vi "HitrapGUI.constructor.vi"(0 "name":string, 2 "data in":string, 5 "error in (no error)":errorcluster) -> (14 "i ref out":refnum<vi>, 16 "data out":string, 19 "error out":errorcluster)   [LabVIEW 2014, in "HitrapGUI.lvlib"]
doc: "This is the constructor of a class.\n\nLicense Agreement for this software:\n\nCopyright (C)\nGesellschaft für Schwerionenforschung, GSI\nPlanckstr. 1\n64291 Darmstadt\nGermany\n\nContact: D.Beck@gsi.de \n\nThis program is free software; you can redistribute it and/or modify it under the terms of the \nGNU General Public License as published by the Free Software Foundation; either version 2 of \nthe license, or (at your option) any later version.\n\nThis program is distributed in the hope that it will be useful, but WITHOUT ANY WARRANTY; \nwithout even the implied warranty of MERCHANTABILITY or FITNESS FOR A PARTICULAR PURPOSE. See the GNU General License for more details (http://www.gnu.org).\n\nGesellschaft für Schwerionenforschung, GSI\nPlanckstr. 1, 64291 Darmstadt, Germany\nFor all questions and ideas contact: M.Richter@gsi.de, H.Brand@gsi.de or D.Beck@gsi.de.\nLast update: 16-JUN-2004"
uses:
  HitrapGUI.lvlib
  CS_Core/CSSystem/CoreLib/CoreLib.byte array 2 string.vi
  CS_Core/GUIs/GOGControllerGUI/GOGControllerGUI.lvlib
  CS_Core/CSSystem/CSSystemLib/CSSystemLib.lvlib
  CS_Core/BaseProcess/BaseProcess.lvlib
  CS_Core/CSSystem/CoreLib/CoreLib.lvlib
  CSlibraries-extern/DimLVEvent/LVDimInterface/LVDimInterface.lvlib
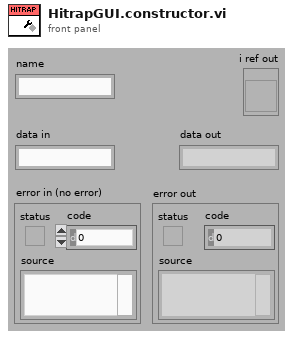
[diagram p1: front panel]
types:
  T1 = enum16{"SetAttribute", "GetAttribute", "CreateAttribute", "DestroyAttribute", "DestroyAllAtributes"}
  T2 = typedef "BaseProcess.lvlib/BaseProcess.i attribute.ctl" = cluster{"EventStatus":string, "EventError":i32, "PresetEvtWatchD":i32, "PresetPdcWatchD":i32, "EventTimeout":i32, "PeriodicInterval":i32, "Interface":string[], "Address":string[], "Special":string[], "PeriodicError":i32, "PeriodicStatus":string, "SuperProc":string, "Descriptors":T3[], "CaseRef":refnum<vi>, "PdcRef":refnum<vi>, "Thread Ref":refnum<vi>, "eventErrorID":i32, "eventStatusID":i32, "periodicErrorID":i32, "periodicStatusID":i32, "pdcCtrID":i32}
  T3 = typedef "BaseProcess.lvlib/BaseProcess.descriptor definition.ctl" = cluster{"selector":string, "descriptor":T4}
  T4 = typedef "BaseProcess.lvlib/BaseProcess.descriptor string definition.ctl" = string
  T5 = typedef "CoreDefs.call_type.ctl" = cluster{"Object":string, "Selector":string, "CallType":enum16{"simple", "synchronous", "asynchronous"}, "Async Object":string, "Async Selector":string, "Data Descriptor":T4, "Data":T6, "Error #":i32, "Expire":u32}
  T6 = typedef "CoreDefs.rawDataType.ctl" = i8[]
  T7 = typedef "HitrapGUI.lvlib/HitrapGUI.i attribute.ctl" = cluster{"SVs":refnum<k21>[], "DSCIntProc":string, "MotorActivityID":i32}
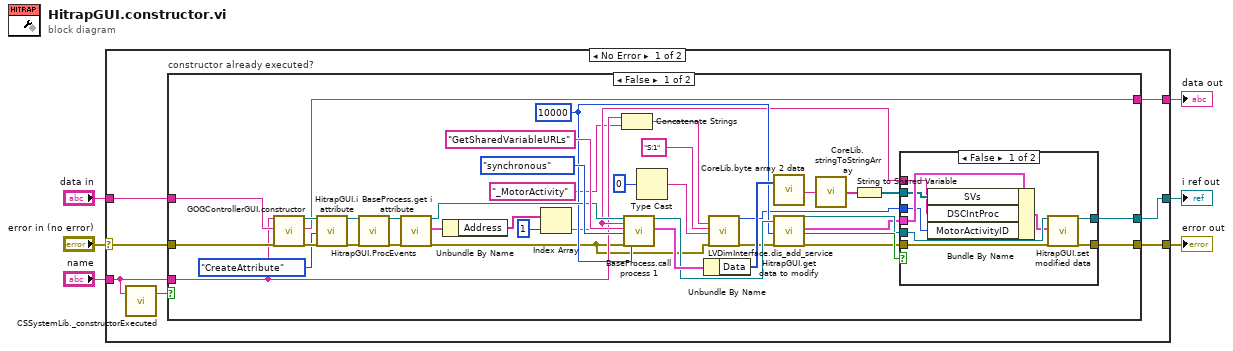
[diagram p0: block diagram]
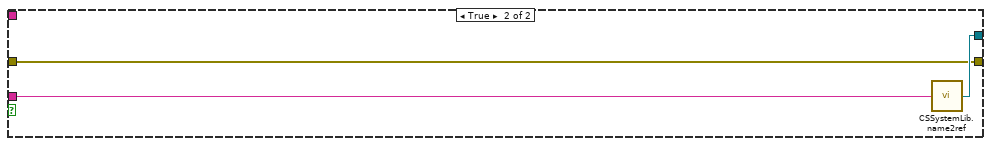
[diagram p3: hidden frame]
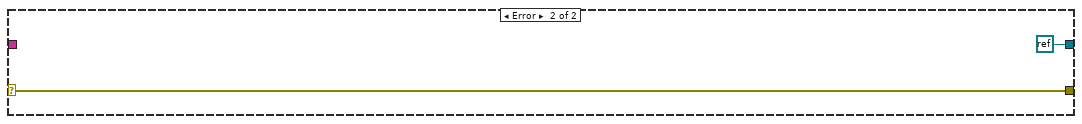
[diagram p4: hidden frame]
diagram:
  n1 = case shown="No Error" "error in (no error)" {
    selector: "error in (no error)" -> [w11 w67]
    tunnel: "name" -> [w10 _]
    tunnel: [w13 refnum<k0> refnum] -> w5
    tunnel: [w12 w67] -> w4
    tunnel: "data in" -> [w8 _]
    tunnel: [w7 _] -> w1
    frame No Error {
      n2 = call "CSSystemLib._constructorExecuted.vi"("name"=w10) -> ("constructor executed?"=w9:bool)  [unwired: 18 in]
      n3 = case "constructor already executed?" shown="False" w9 {
        tunnel: w10 -> [w19 w66]
        tunnel: [w29 w65] -> w13
        tunnel: [w27 w64] -> w12
        tunnel: w11 -> [w47 w64]
        tunnel: w8 -> [w46 _]
        tunnel: [w45 _] -> w7
        frame False {
          w32 = 10000 ("timeout (ms)")
          n4 = call "GOGControllerGUI.constructor.vi"("name"=w19, "data in"=w46, "error in (no error)"=w47) -> ("i ref out"=w52:refnum<vi>, "data out"=w45:string, "error out"=w51:errorcluster)  [unwired: 14 in]
          n5 = call "HitrapGUI.i attribute.vi"("VI Refnum"=w52, "Action"=T1."CreateAttribute", "error in (no error)"=w51) -> ("VI Refnum out"=w49:refnum<vi>, "error out"=w48:errorcluster)  [unwired: 14 in, 1 out]
          n6 = call "HitrapGUI.ProcEvents.vi"("i ref in"=w49, "error in (no error)"=w48) -> ("i ref out"=w34:refnum<vi>, "error out"=w35:errorcluster)  [unwired: 16 in]
          n7 = call "BaseProcess.get i attribute.vi"("i ref in"=w34, "error in (no error)"=w35) -> ("i ref out"=w36:refnum<vi>, "i attribute"=w44:T2, "error out"=w14:errorcluster)  [unwired: 15 in]
          n8 = Unbundle By Name(w44) -> ("Address"=w43:string[])
          n9 = Index Array(array=w43, index=1) -> (element=w23:string)
          n10 = Concatenate Strings(w19, "_MotorActivity" ("string")) -> (w20:string)
          n11 = call "BaseProcess.call process 1.vi"("i ref in"=w36, "Object"=w23, "Selector"="GetSharedVariableURLs", "CallType"=enum16{"simple", "synchronous", "asynchronous"}."synchronous", "error in (no error)"=w14, "timeout (ms)"=w32) -> ("i ref out"=w33:refnum<vi>, "call cluster out"=w39:T5)  [unwired: 11 in, 1 out]
          n12 = Type Cast(x=i16 0) -> (*(type *) &x=w15:string)  [unwired: 1 in]
          n13 = Unbundle By Name(w39) -> ("Data"=w40:T6)
          n14 = call "LVDimInterface.dis_add_service.vi"("serviceName"=w20, "typeDescriptor"="S:1", "data"=w15, "error in (no error)"=w14) -> ("my_serviceID"=w22:i32, "error out"=w21:errorcluster)  [unwired: 14 in]
          n15 = call-poly "CoreLib.byte array 2 data.vi"("byteArray"=w40) -> ("string"=w41:string)  [unwired: 16 in, 2 out]
          n16 = call "HitrapGUI.get data to modify.vi"("i ref in"=w33, "ms timeout (10000)"=w32, "error in (no error)"=w21) -> ("i ref out"=w30:refnum<vi>, "i attribute"=w26:T7, "timed out"=w31:bool, "error out"=w28:errorcluster)  [unwired: 13 in]
          n17 = call "CoreLib.stringToStringArray.vi"("String"=w41) -> ("Array"=w25:string[])
          n18 = String to Shared Variable(0:w25) -> (2:w24:refnum<k21>[])  [unwired: 1 out]
          n19 = case shown="False" w31 {
            tunnel: w30 -> [w61 w63]
            tunnel: [w60 w63] -> w29
            tunnel: w28 -> [w59 w62]
            tunnel: [w58 w62] -> w27
            tunnel: w26 -> [w57 _]
            tunnel: w24 -> [w55 _]
            tunnel: w23 -> [w54 _]
            tunnel: w22 -> [w53 _]
            frame False {
              n20 = Bundle By Name(cluster=w57, "SVs"=w55, "DSCIntProc"=w54, "MotorActivityID"=w53) -> (w56:T7)
              n21 = call "HitrapGUI.set modified data.vi"("i ref in"=w61, "i attribute"=w56, "error in (no error)"=w59) -> ("i ref out"=w60:refnum<vi>, "error out"=w58:errorcluster)  [unwired: 15 in]
            }
            frame True {
            }
          }
        }
        frame True {
          n22 = call "CSSystemLib.name2ref.vi"("name"=w66) -> ("obj refnum"=w65:refnum<vi>)
        }
      }
    }
    frame Error {
    }
  }
  "i ref out" <- w5
  "error out" <- w4
  "data out" <- w1
